vi "UTILITY Modbus Boolean Bit Flip.vi"(11 "Input WORD":u16 format="%x") -> (3 "Flipped Bytes (16 bits)":bool[](array[boolean]))   [LabVIEW 2016]
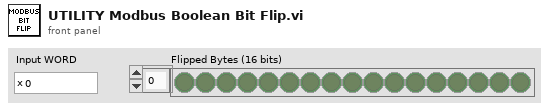
[diagram p1: front panel]
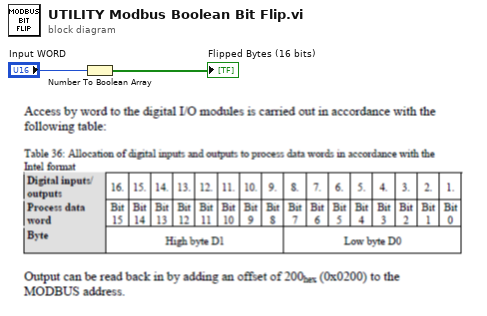
[diagram p0: block diagram]
diagram:
  n1 = Number To Boolean Array(number="Input WORD") -> (Boolean array=→"Flipped Bytes (16 bits)":bool[])
